vi "Initialize Close Variables.vi"(7 "Action":enum16{"Init", "Close"}(ring)=enum."Close", 8 "error in (no error)":errorcluster) -> (0 "error out":errorcluster)   [LabVIEW 2019]
uses:
  Controls/UDP - Event.ctl
  Controls/UDP - Status.ctl
  Controls/eFGV States.ctl
  Controls/FGV States.ctl
  Controls/Global - Device.vi
  Controls/Global - IP Address.vi
  Controls/Global - Done.vi
  Controls/Global - Comport.vi
  Controls/Global - Handle.vi
  Controls/Global - Unit.vi
  Controls/Global - ADC.vi
  Controls/Global - PID.vi
  Controls/Global - System.vi
  Controls/Global - Test.vi
  Controls/Global - Channel.vi
  Controls/Global - Data UDP.vi
  Controls/Global - Rendezvous.vi
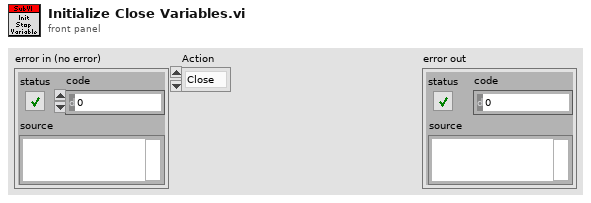
[diagram p1: front panel]
types:
  T1 = cluster{"Ch1":sgl, "Ch2":sgl, "Ch3":sgl, "Ch4":sgl, "Ch5":sgl, "Ch6":sgl, "Ch7":sgl, "Ch8":sgl, "Ch9":sgl, "Ch10":sgl, "Ch11":sgl, "Ch12":sgl, "Ch13":sgl, "Ch14":sgl, "Ch15":sgl, "Ch16":sgl}
  T2 = typedef "UDP - Event.ctl" = u16
  T3 = typedef "UDP - Status.ctl" = u16
  T4 = cluster{"Channels":cluster{"Ch1":sgl, "Ch2":sgl, "Ch3":sgl, "Ch4":sgl, "Ch5":sgl, "Ch6":sgl, "Ch7":sgl, "Ch8":sgl, "Ch9":sgl, "Ch10":sgl, "Ch11":sgl, "Ch12":sgl, "Ch13":sgl, "Ch14":sgl, "Ch15":sgl, "Ch16":sgl}, "Event":T2, "Status":T3, "IP":string}[]
  T5 = cluster{"Target Load":sgl, "Target Disp":sgl, "Rate":sgl, "Speed":sgl}[]
  T6 = cluster{"Out Type":u8, "Inverse":u8, "Monitor":u8, "Reserve":u8, "ACC Time":u32, "Pulse Rev":u32, "Stroke":u32, "Auto Off":u32, "Gear Ratio":sgl, "Pitch":sgl, "Max Speed":u32, "Jog Speed":u32, "Disp Coff":sgl, "Max Load":u32}[]
  T7 = cluster{"SP":sgl, "PV":sgl, "kP":sgl, "kI":sgl, "kD":sgl, "FF":sgl, "Err Band":sgl, "Max":i32, "Min":i32, "Ts":u32, "Out":i32, "Mode":u8}[]
  T8 = cluster{"Active Ch":u8[], "Filter Type":u8, "Post Filter":u8[], "Gain":u8[], "FS":u16, "IntOC":u8, "IntFC":u8, "SysOC":u8, "Cofficient":dbl[], "K":dbl[], "Max":i32}[]
  T9 = cluster{"Name":string[], "Unit":string[], "Decimal Point":u8[], "Ch Log":u8[], "H Alarm":u8[], "L Alarm":u8[], "H Limit":sgl[], "L Limit":sgl[], "Filter":u8[], "Gain":u8[], "Calib Type":u32[]}[]
  T10 = cluster{"IP Address":string, "port":string, "UDP ref":refnum<k16>}[]
  T11 = typedef "FGV States.ctl" = enum16{"Read", "Write"}
  T12 = typedef "eFGV States.ctl" = enum16{"Init", "Read", "Write", "Exit"}
  T13 = typedef "Rendezvous RefNum" = refnum<k1>
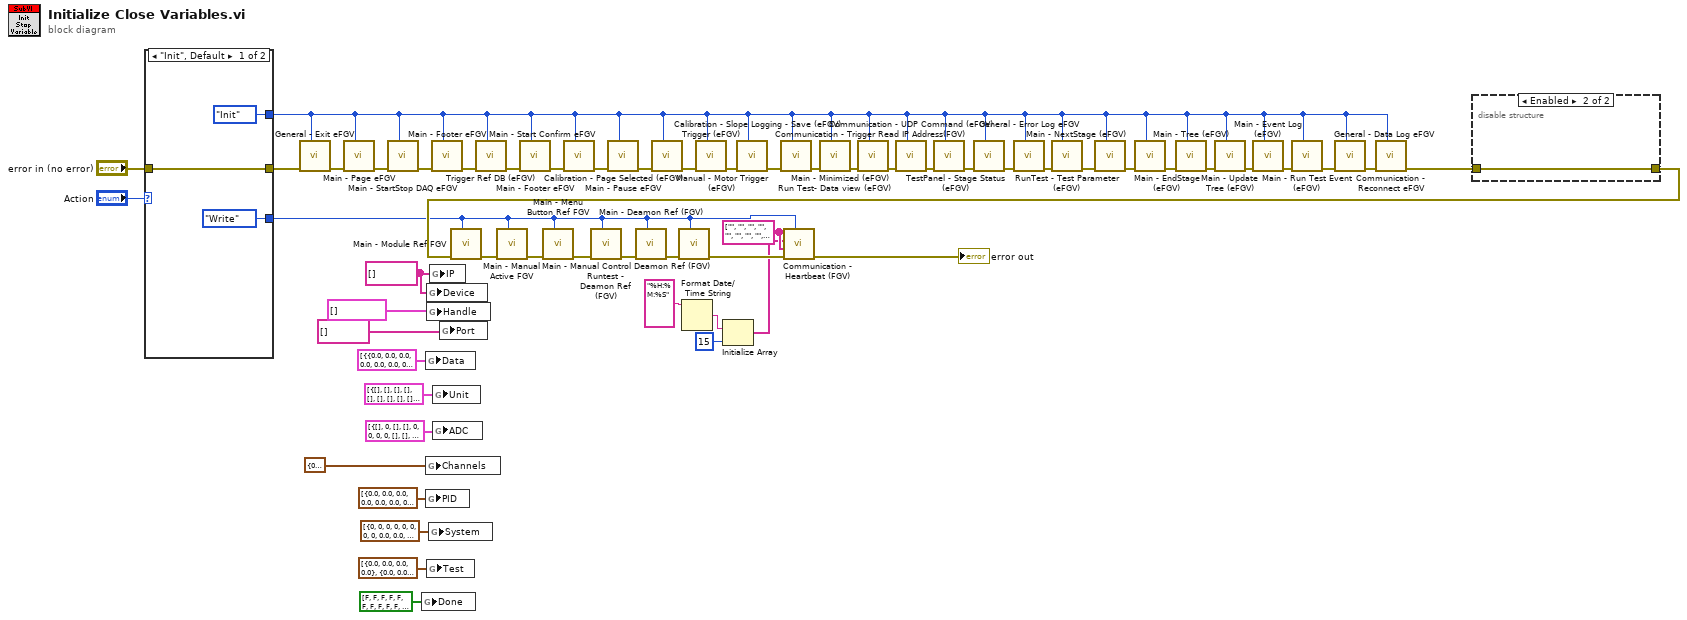
[diagram p0: block diagram]
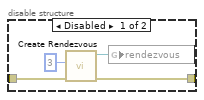
[diagram p2: hidden frame]
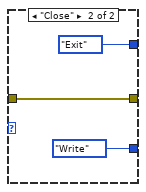
[diagram p3: hidden frame]
diagram:
  w10 = string[] ["", "", "", "", "", "", "", "", "", "", "", "", "", "", "", ""] ("IP")
  w35 = string[] [] ("SN")
  n1 = case shown="\"Init\", Default" "Action" {
    tunnel: [eFGV_States."Init" ("eFGV States") eFGV_States."Exit" ("eFGV States")] -> w1
    tunnel: [w58 w61] -> w55
    tunnel: "error in (no error)" -> [w58 w61]
    tunnel: [FGV_States."Write" ("Action") FGV_States."Write" ("Action")] -> w11
    frame "Init", Default {
    }
    frame "Close" {
    }
  }
  n2 = call "General - Exit eFGV.vi"("eFGV States"=w1, "error in (no error)"=w55) -> ("error out"=w48:errorcluster)  [unwired: 7 in, 2 out]
  n3 = call "Main - Page eFGV.vi"("eFGV States"=w1, "error in (no error)"=w48) -> ("error out"=w47:errorcluster)  [unwired: 7 in, 2 out]
  n4 = call "Main - StartStop DAQ eFGV.vi"("Action"=w1, "error in"=w47) -> ("error out"=w53:errorcluster)  [unwired: 7 in, 2 out]
  n5 = global write "Global - Done.vi" "Done"(bool[] [FALSE, FALSE, FALSE, FALSE, FALSE, FALSE, FALSE, FALSE, FALSE, FALSE, FALSE, FALSE, FALSE, FALSE, FALSE, FALSE] ("Done")) -> ()
  n6 = global write "Global - Channel.vi" "Data"(T4 [{"Channels"={"Ch1"=0.0, "Ch2"=0.0, "Ch3"=0.0, "Ch4"=0.0, "Ch5"=0.0, "Ch6"=0.0, "Ch7"=0.0, "Ch8"=0.0, "Ch9"=0.0, "Ch10"=0.0, "Ch11"=0.0, "Ch12"=0.0, "Ch13"=0.0, "Ch14"=0.0, "Ch15"=0.0, "Ch16"=0.0}, "Event"=0, "Status"=0, "IP"=""}, {"Channels"={"Ch1"=0.0, "Ch2"=0.0, "Ch3"=0.0, "Ch4"=0.0, "Ch5"=0.0, "Ch6"=0.0, "Ch7"=0.0, "Ch8"=0.0, "Ch9"=0.0, "Ch10"=0.0, "Ch11"=0.0, "Ch12"=0.0, "Ch13"=0.0, "Ch14"=0.0, "Ch15"=0.0, "Ch16"=0.0}, "Event"=0, "Status"=0, "IP"=""}, {"Channels"={"Ch1"=0.0, "Ch2"=0.0, "Ch3"=0.0, "Ch4"=0.0, "Ch5"=0.0, "Ch6"=0.0, "Ch7"=0.0, "Ch8"=0.0, "Ch9"=0.0, "Ch10"=0.0, "Ch11"=0.0, "Ch12"=0.0, "Ch13"=0.0, "Ch14"=0.0, "Ch15"=0.0, "Ch16"=0.0}, "Event"=0, "Status"=0, "IP"=""}, {"Channels"={"Ch1"=0.0, "Ch2"=0.0, "Ch3"=0.0, "Ch4"=0.0, "Ch5"=0.0, "Ch6"=0.0, "Ch7"=0.0, "Ch8"=0.0, "Ch9"=0.0, "Ch10"=0.0, "Ch11"=0.0, "Ch12"=0.0, "Ch13"=0.0, "Ch14"=0.0, "Ch15"=0.0, "Ch16"=0.0}, "Event"=0, "Status"=0, "IP"=""}, {"Channels"={"Ch1"=0.0, "Ch2"=0.0, "Ch3"=0.0, "Ch4"=0.0, "Ch5"=0.0, "Ch6"=0.0, "Ch7"=0.0, "Ch8"=0.0, "Ch9"=0.0, "Ch10"=0.0, "Ch11"=0.0, "Ch12"=0.0, "Ch13"=0.0, "Ch14"=0.0, "Ch15"=0.0, "Ch16"=0.0}, "Event"=0, "Status"=0, "IP"=""}, {"Channels"={"Ch1"=0.0, "Ch2"=0.0, "Ch3"=0.0, "Ch4"=0.0, "Ch5"=0.0, "Ch6"=0.0, "Ch7"=0.0, "Ch8"=0.0, "Ch9"=0.0, "Ch10"=0.0, "Ch11"=0.0, "Ch12"=0.0, "Ch13"=0.0, "Ch14"=0.0, "Ch15"=0.0, "Ch16"=0.0}, "Event"=0, "Status"=0, "IP"=""}, {"Channels"={"Ch1"=0.0, "Ch2"=0.0, "Ch3"=0.0, "Ch4"=0.0, "Ch5"=0.0, "Ch6"=0.0, "Ch7"=0.0, "Ch8"=0.0, "Ch9"=0.0, "Ch10"=0.0, "Ch11"=0.0, "Ch12"=0.0, "Ch13"=0.0, "Ch14"=0.0, "Ch15"=0.0, "Ch16"=0.0}, "Event"=0, "Status"=0, "IP"=""}, {"Channels"={"Ch1"=0.0, "Ch2"=0.0, "Ch3"=0.0, "Ch4"=0.0, "Ch5"=0.0, "Ch6"=0.0, "Ch7"=0.0, "Ch8"=0.0, "Ch9"=0.0, "Ch10"=0.0, "Ch11"=0.0, "Ch12"=0.0, "Ch13"=0.0, "Ch14"=0.0, "Ch15"=0.0, "Ch16"=0.0}, "Event"=0, "Status"=0, "IP"=""}, {"Channels"={"Ch1"=0.0, "Ch2"=0.0, "Ch3"=0.0, "Ch4"=0.0, "Ch5"=0.0, "Ch6"=0.0, "Ch7"=0.0, "Ch8"=0.0, "Ch9"=0.0, "Ch10"=0.0, "Ch11"=0.0, "Ch12"=0.0, "Ch13"=0.0, "Ch14"=0.0, "Ch15"=0.0, "Ch16"=0.0}, "Event"=0, "Status"=0, "IP"=""}, {"Channels"={"Ch1"=0.0, "Ch2"=0.0, "Ch3"=0.0, "Ch4"=0.0, "Ch5"=0.0, "Ch6"=0.0, "Ch7"=0.0, "Ch8"=0.0, "Ch9"=0.0, "Ch10"=0.0, "Ch11"=0.0, "Ch12"=0.0, "Ch13"=0.0, "Ch14"=0.0, "Ch15"=0.0, "Ch16"=0.0}, "Event"=0, "Status"=0, "IP"=""}, {"Channels"={"Ch1"=0.0, "Ch2"=0.0, "Ch3"=0.0, "Ch4"=0.0, "Ch5"=0.0, "Ch6"=0.0, "Ch7"=0.0, "Ch8"=0.0, "Ch9"=0.0, "Ch10"=0.0, "Ch11"=0.0, "Ch12"=0.0, "Ch13"=0.0, "Ch14"=0.0, "Ch15"=0.0, "Ch16"=0.0}, "Event"=0, "Status"=0, "IP"=""}, {"Channels"={"Ch1"=0.0, "Ch2"=0.0, "Ch3"=0.0, "Ch4"=0.0, "Ch5"=0.0, "Ch6"=0.0, "Ch7"=0.0, "Ch8"=0.0, "Ch9"=0.0, "Ch10"=0.0, "Ch11"=0.0, "Ch12"=0.0, "Ch13"=0.0, "Ch14"=0.0, "Ch15"=0.0, "Ch16"=0.0}, "Event"=0, "Status"=0, "IP"=""}, {"Channels"={"Ch1"=0.0, "Ch2"=0.0, "Ch3"=0.0, "Ch4"=0.0, "Ch5"=0.0, "Ch6"=0.0, "Ch7"=0.0, "Ch8"=0.0, "Ch9"=0.0, "Ch10"=0.0, "Ch11"=0.0, "Ch12"=0.0, "Ch13"=0.0, "Ch14"=0.0, "Ch15"=0.0, "Ch16"=0.0}, "Event"=0, "Status"=0, "IP"=""}, {"Channels"={"Ch1"=0.0, "Ch2"=0.0, "Ch3"=0.0, "Ch4"=0.0, "Ch5"=0.0, "Ch6"=0.0, "Ch7"=0.0, "Ch8"=0.0, "Ch9"=0.0, "Ch10"=0.0, "Ch11"=0.0, "Ch12"=0.0, "Ch13"=0.0, "Ch14"=0.0, "Ch15"=0.0, "Ch16"=0.0}, "Event"=0, "Status"=0, "IP"=""}, {"Channels"={"Ch1"=0.0, "Ch2"=0.0, "Ch3"=0.0, "Ch4"=0.0, "Ch5"=0.0, "Ch6"=0.0, "Ch7"=0.0, "Ch8"=0.0, "Ch9"=0.0, "Ch10"=0.0, "Ch11"=0.0, "Ch12"=0.0, "Ch13"=0.0, "Ch14"=0.0, "Ch15"=0.0, "Ch16"=0.0}, "Event"=0, "Status"=0, "IP"=""}, {"Channels"={"Ch1"=0.0, "Ch2"=0.0, "Ch3"=0.0, "Ch4"=0.0, "Ch5"=0.0, "Ch6"=0.0, "Ch7"=0.0, "Ch8"=0.0, "Ch9"=0.0, "Ch10"=0.0, "Ch11"=0.0, "Ch12"=0.0, "Ch13"=0.0, "Ch14"=0.0, "Ch15"=0.0, "Ch16"=0.0}, "Event"=0, "Status"=0, "IP"=""}] ("Data")) -> ()
  n7 = global write "Global - Data UDP.vi" "Channels"(T1 {"Ch1"=0.0, "Ch2"=0.0, "Ch3"=0.0, "Ch4"=0.0, "Ch5"=0.0, "Ch6"=0.0, "Ch7"=0.0, "Ch8"=0.0, "Ch9"=0.0, "Ch10"=0.0, "Ch11"=0.0, "Ch12"=0.0, "Ch13"=0.0, "Ch14"=0.0, "Ch15"=0.0, "Ch16"=0.0} ("Channels")) -> ()
  n8 = global write "Global - PID.vi" "PID"(T7 [{"SP"=0.0, "PV"=0.0, "kP"=0.0, "kI"=0.0, "kD"=0.0, "FF"=0.0, "Err Band"=0.0, "Max"=0, "Min"=0, "Ts"=0, "Out"=0, "Mode"=0}, {"SP"=0.0, "PV"=0.0, "kP"=0.0, "kI"=0.0, "kD"=0.0, "FF"=0.0, "Err Band"=0.0, "Max"=0, "Min"=0, "Ts"=0, "Out"=0, "Mode"=0}, {"SP"=0.0, "PV"=0.0, "kP"=0.0, "kI"=0.0, "kD"=0.0, "FF"=0.0, "Err Band"=0.0, "Max"=0, "Min"=0, "Ts"=0, "Out"=0, "Mode"=0}, {"SP"=0.0, "PV"=0.0, "kP"=0.0, "kI"=0.0, "kD"=0.0, "FF"=0.0, "Err Band"=0.0, "Max"=0, "Min"=0, "Ts"=0, "Out"=0, "Mode"=0}, {"SP"=0.0, "PV"=0.0, "kP"=0.0, "kI"=0.0, "kD"=0.0, "FF"=0.0, "Err Band"=0.0, "Max"=0, "Min"=0, "Ts"=0, "Out"=0, "Mode"=0}, {"SP"=0.0, "PV"=0.0, "kP"=0.0, "kI"=0.0, "kD"=0.0, "FF"=0.0, "Err Band"=0.0, "Max"=0, "Min"=0, "Ts"=0, "Out"=0, "Mode"=0}, {"SP"=0.0, "PV"=0.0, "kP"=0.0, "kI"=0.0, "kD"=0.0, "FF"=0.0, "Err Band"=0.0, "Max"=0, "Min"=0, "Ts"=0, "Out"=0, "Mode"=0}, {"SP"=0.0, "PV"=0.0, "kP"=0.0, "kI"=0.0, "kD"=0.0, "FF"=0.0, "Err Band"=0.0, "Max"=0, "Min"=0, "Ts"=0, "Out"=0, "Mode"=0}, {"SP"=0.0, "PV"=0.0, "kP"=0.0, "kI"=0.0, "kD"=0.0, "FF"=0.0, "Err Band"=0.0, "Max"=0, "Min"=0, "Ts"=0, "Out"=0, "Mode"=0}, {"SP"=0.0, "PV"=0.0, "kP"=0.0, "kI"=0.0, "kD"=0.0, "FF"=0.0, "Err Band"=0.0, "Max"=0, "Min"=0, "Ts"=0, "Out"=0, "Mode"=0}, {"SP"=0.0, "PV"=0.0, "kP"=0.0, "kI"=0.0, "kD"=0.0, "FF"=0.0, "Err Band"=0.0, "Max"=0, "Min"=0, "Ts"=0, "Out"=0, "Mode"=0}, {"SP"=0.0, "PV"=0.0, "kP"=0.0, "kI"=0.0, "kD"=0.0, "FF"=0.0, "Err Band"=0.0, "Max"=0, "Min"=0, "Ts"=0, "Out"=0, "Mode"=0}, {"SP"=0.0, "PV"=0.0, "kP"=0.0, "kI"=0.0, "kD"=0.0, "FF"=0.0, "Err Band"=0.0, "Max"=0, "Min"=0, "Ts"=0, "Out"=0, "Mode"=0}, {"SP"=0.0, "PV"=0.0, "kP"=0.0, "kI"=0.0, "kD"=0.0, "FF"=0.0, "Err Band"=0.0, "Max"=0, "Min"=0, "Ts"=0, "Out"=0, "Mode"=0}, {"SP"=0.0, "PV"=0.0, "kP"=0.0, "kI"=0.0, "kD"=0.0, "FF"=0.0, "Err Band"=0.0, "Max"=0, "Min"=0, "Ts"=0, "Out"=0, "Mode"=0}, {"SP"=0.0, "PV"=0.0, "kP"=0.0, "kI"=0.0, "kD"=0.0, "FF"=0.0, "Err Band"=0.0, "Max"=0, "Min"=0, "Ts"=0, "Out"=0, "Mode"=0}] ("PID")) -> ()
  n9 = global write "Global - Device.vi" "Device"(w35) -> ()
  n10 = global write "Global - Handle.vi" "Handle"(T10 [] ("Handle")) -> ()
  n11 = global write "Global - Test.vi" "Test"(T5 [{"Target Load"=0.0, "Target Disp"=0.0, "Rate"=0.0, "Speed"=0.0}, {"Target Load"=0.0, "Target Disp"=0.0, "Rate"=0.0, "Speed"=0.0}, {"Target Load"=0.0, "Target Disp"=0.0, "Rate"=0.0, "Speed"=0.0}, {"Target Load"=0.0, "Target Disp"=0.0, "Rate"=0.0, "Speed"=0.0}, {"Target Load"=0.0, "Target Disp"=0.0, "Rate"=0.0, "Speed"=0.0}, {"Target Load"=0.0, "Target Disp"=0.0, "Rate"=0.0, "Speed"=0.0}, {"Target Load"=0.0, "Target Disp"=0.0, "Rate"=0.0, "Speed"=0.0}, {"Target Load"=0.0, "Target Disp"=0.0, "Rate"=0.0, "Speed"=0.0}, {"Target Load"=0.0, "Target Disp"=0.0, "Rate"=0.0, "Speed"=0.0}, {"Target Load"=0.0, "Target Disp"=0.0, "Rate"=0.0, "Speed"=0.0}, {"Target Load"=0.0, "Target Disp"=0.0, "Rate"=0.0, "Speed"=0.0}, {"Target Load"=0.0, "Target Disp"=0.0, "Rate"=0.0, "Speed"=0.0}, {"Target Load"=0.0, "Target Disp"=0.0, "Rate"=0.0, "Speed"=0.0}, {"Target Load"=0.0, "Target Disp"=0.0, "Rate"=0.0, "Speed"=0.0}, {"Target Load"=0.0, "Target Disp"=0.0, "Rate"=0.0, "Speed"=0.0}, {"Target Load"=0.0, "Target Disp"=0.0, "Rate"=0.0, "Speed"=0.0}] ("Test")) -> ()
  n12 = global write "Global - System.vi" "System"(T6 [{"Out Type"=0, "Inverse"=0, "Monitor"=0, "Reserve"=0, "ACC Time"=0, "Pulse Rev"=0, "Stroke"=0, "Auto Off"=0, "Gear Ratio"=0.0, "Pitch"=0.0, "Max Speed"=0, "Jog Speed"=0, "Disp Coff"=0.0, "Max Load"=0}, {"Out Type"=0, "Inverse"=0, "Monitor"=0, "Reserve"=0, "ACC Time"=0, "Pulse Rev"=0, "Stroke"=0, "Auto Off"=0, "Gear Ratio"=0.0, "Pitch"=0.0, "Max Speed"=0, "Jog Speed"=0, "Disp Coff"=0.0, "Max Load"=0}, {"Out Type"=0, "Inverse"=0, "Monitor"=0, "Reserve"=0, "ACC Time"=0, "Pulse Rev"=0, "Stroke"=0, "Auto Off"=0, "Gear Ratio"=0.0, "Pitch"=0.0, "Max Speed"=0, "Jog Speed"=0, "Disp Coff"=0.0, "Max Load"=0}, {"Out Type"=0, "Inverse"=0, "Monitor"=0, "Reserve"=0, "ACC Time"=0, "Pulse Rev"=0, "Stroke"=0, "Auto Off"=0, "Gear Ratio"=0.0, "Pitch"=0.0, "Max Speed"=0, "Jog Speed"=0, "Disp Coff"=0.0, "Max Load"=0}, {"Out Type"=0, "Inverse"=0, "Monitor"=0, "Reserve"=0, "ACC Time"=0, "Pulse Rev"=0, "Stroke"=0, "Auto Off"=0, "Gear Ratio"=0.0, "Pitch"=0.0, "Max Speed"=0, "Jog Speed"=0, "Disp Coff"=0.0, "Max Load"=0}, {"Out Type"=0, "Inverse"=0, "Monitor"=0, "Reserve"=0, "ACC Time"=0, "Pulse Rev"=0, "Stroke"=0, "Auto Off"=0, "Gear Ratio"=0.0, "Pitch"=0.0, "Max Speed"=0, "Jog Speed"=0, "Disp Coff"=0.0, "Max Load"=0}, {"Out Type"=0, "Inverse"=0, "Monitor"=0, "Reserve"=0, "ACC Time"=0, "Pulse Rev"=0, "Stroke"=0, "Auto Off"=0, "Gear Ratio"=0.0, "Pitch"=0.0, "Max Speed"=0, "Jog Speed"=0, "Disp Coff"=0.0, "Max Load"=0}, {"Out Type"=0, "Inverse"=0, "Monitor"=0, "Reserve"=0, "ACC Time"=0, "Pulse Rev"=0, "Stroke"=0, "Auto Off"=0, "Gear Ratio"=0.0, "Pitch"=0.0, "Max Speed"=0, "Jog Speed"=0, "Disp Coff"=0.0, "Max Load"=0}, {"Out Type"=0, "Inverse"=0, "Monitor"=0, "Reserve"=0, "ACC Time"=0, "Pulse Rev"=0, "Stroke"=0, "Auto Off"=0, "Gear Ratio"=0.0, "Pitch"=0.0, "Max Speed"=0, "Jog Speed"=0, "Disp Coff"=0.0, "Max Load"=0}, {"Out Type"=0, "Inverse"=0, "Monitor"=0, "Reserve"=0, "ACC Time"=0, "Pulse Rev"=0, "Stroke"=0, "Auto Off"=0, "Gear Ratio"=0.0, "Pitch"=0.0, "Max Speed"=0, "Jog Speed"=0, "Disp Coff"=0.0, "Max Load"=0}, {"Out Type"=0, "Inverse"=0, "Monitor"=0, "Reserve"=0, "ACC Time"=0, "Pulse Rev"=0, "Stroke"=0, "Auto Off"=0, "Gear Ratio"=0.0, "Pitch"=0.0, "Max Speed"=0, "Jog Speed"=0, "Disp Coff"=0.0, "Max Load"=0}, {"Out Type"=0, "Inverse"=0, "Monitor"=0, "Reserve"=0, "ACC Time"=0, "Pulse Rev"=0, "Stroke"=0, "Auto Off"=0, "Gear Ratio"=0.0, "Pitch"=0.0, "Max Speed"=0, "Jog Speed"=0, "Disp Coff"=0.0, "Max Load"=0}, {"Out Type"=0, "Inverse"=0, "Monitor"=0, "Reserve"=0, "ACC Time"=0, "Pulse Rev"=0, "Stroke"=0, "Auto Off"=0, "Gear Ratio"=0.0, "Pitch"=0.0, "Max Speed"=0, "Jog Speed"=0, "Disp Coff"=0.0, "Max Load"=0}, {"Out Type"=0, "Inverse"=0, "Monitor"=0, "Reserve"=0, "ACC Time"=0, "Pulse Rev"=0, "Stroke"=0, "Auto Off"=0, "Gear Ratio"=0.0, "Pitch"=0.0, "Max Speed"=0, "Jog Speed"=0, "Disp Coff"=0.0, "Max Load"=0}, {"Out Type"=0, "Inverse"=0, "Monitor"=0, "Reserve"=0, "ACC Time"=0, "Pulse Rev"=0, "Stroke"=0, "Auto Off"=0, "Gear Ratio"=0.0, "Pitch"=0.0, "Max Speed"=0, "Jog Speed"=0, "Disp Coff"=0.0, "Max Load"=0}, {"Out Type"=0, "Inverse"=0, "Monitor"=0, "Reserve"=0, "ACC Time"=0, "Pulse Rev"=0, "Stroke"=0, "Auto Off"=0, "Gear Ratio"=0.0, "Pitch"=0.0, "Max Speed"=0, "Jog Speed"=0, "Disp Coff"=0.0, "Max Load"=0}] ("System")) -> ()
  n13 = global write "Global - IP Address.vi" "IP"(w35) -> ()
  n14 = call "Main - Footer eFGV.vi"("Action"=w1, "error in"=w53) -> ("error out"=w46:errorcluster)  [unwired: 7 in, 2 out]
  n15 = global write "Global - Unit.vi" "Unit"(T9 [{"Name"=[], "Unit"=[], "Decimal Point"=[], "Ch Log"=[], "H Alarm"=[], "L Alarm"=[], "H Limit"=[], "L Limit"=[], "Filter"=[], "Gain"=[], "Calib Type"=[]}, {"Name"=[], "Unit"=[], "Decimal Point"=[], "Ch Log"=[], "H Alarm"=[], "L Alarm"=[], "H Limit"=[], "L Limit"=[], "Filter"=[], "Gain"=[], "Calib Type"=[]}, {"Name"=[], "Unit"=[], "Decimal Point"=[], "Ch Log"=[], "H Alarm"=[], "L Alarm"=[], "H Limit"=[], "L Limit"=[], "Filter"=[], "Gain"=[], "Calib Type"=[]}, {"Name"=[], "Unit"=[], "Decimal Point"=[], "Ch Log"=[], "H Alarm"=[], "L Alarm"=[], "H Limit"=[], "L Limit"=[], "Filter"=[], "Gain"=[], "Calib Type"=[]}, {"Name"=[], "Unit"=[], "Decimal Point"=[], "Ch Log"=[], "H Alarm"=[], "L Alarm"=[], "H Limit"=[], "L Limit"=[], "Filter"=[], "Gain"=[], "Calib Type"=[]}, {"Name"=[], "Unit"=[], "Decimal Point"=[], "Ch Log"=[], "H Alarm"=[], "L Alarm"=[], "H Limit"=[], "L Limit"=[], "Filter"=[], "Gain"=[], "Calib Type"=[]}, {"Name"=[], "Unit"=[], "Decimal Point"=[], "Ch Log"=[], "H Alarm"=[], "L Alarm"=[], "H Limit"=[], "L Limit"=[], "Filter"=[], "Gain"=[], "Calib Type"=[]}, {"Name"=[], "Unit"=[], "Decimal Point"=[], "Ch Log"=[], "H Alarm"=[], "L Alarm"=[], "H Limit"=[], "L Limit"=[], "Filter"=[], "Gain"=[], "Calib Type"=[]}, {"Name"=[], "Unit"=[], "Decimal Point"=[], "Ch Log"=[], "H Alarm"=[], "L Alarm"=[], "H Limit"=[], "L Limit"=[], "Filter"=[], "Gain"=[], "Calib Type"=[]}, {"Name"=[], "Unit"=[], "Decimal Point"=[], "Ch Log"=[], "H Alarm"=[], "L Alarm"=[], "H Limit"=[], "L Limit"=[], "Filter"=[], "Gain"=[], "Calib Type"=[]}, {"Name"=[], "Unit"=[], "Decimal Point"=[], "Ch Log"=[], "H Alarm"=[], "L Alarm"=[], "H Limit"=[], "L Limit"=[], "Filter"=[], "Gain"=[], "Calib Type"=[]}, {"Name"=[], "Unit"=[], "Decimal Point"=[], "Ch Log"=[], "H Alarm"=[], "L Alarm"=[], "H Limit"=[], "L Limit"=[], "Filter"=[], "Gain"=[], "Calib Type"=[]}, {"Name"=[], "Unit"=[], "Decimal Point"=[], "Ch Log"=[], "H Alarm"=[], "L Alarm"=[], "H Limit"=[], "L Limit"=[], "Filter"=[], "Gain"=[], "Calib Type"=[]}, {"Name"=[], "Unit"=[], "Decimal Point"=[], "Ch Log"=[], "H Alarm"=[], "L Alarm"=[], "H Limit"=[], "L Limit"=[], "Filter"=[], "Gain"=[], "Calib Type"=[]}, {"Name"=[], "Unit"=[], "Decimal Point"=[], "Ch Log"=[], "H Alarm"=[], "L Alarm"=[], "H Limit"=[], "L Limit"=[], "Filter"=[], "Gain"=[], "Calib Type"=[]}, {"Name"=[], "Unit"=[], "Decimal Point"=[], "Ch Log"=[], "H Alarm"=[], "L Alarm"=[], "H Limit"=[], "L Limit"=[], "Filter"=[], "Gain"=[], "Calib Type"=[]}] ("Unit")) -> ()
  n16 = global write "Global - ADC.vi" "ADC"(T8 [{"Active Ch"=[], "Filter Type"=0, "Post Filter"=[], "Gain"=[], "FS"=0, "IntOC"=0, "IntFC"=0, "SysOC"=0, "Cofficient"=[], "K"=[], "Max"=0}, {"Active Ch"=[], "Filter Type"=0, "Post Filter"=[], "Gain"=[], "FS"=0, "IntOC"=0, "IntFC"=0, "SysOC"=0, "Cofficient"=[], "K"=[], "Max"=0}, {"Active Ch"=[], "Filter Type"=0, "Post Filter"=[], "Gain"=[], "FS"=0, "IntOC"=0, "IntFC"=0, "SysOC"=0, "Cofficient"=[], "K"=[], "Max"=0}, {"Active Ch"=[], "Filter Type"=0, "Post Filter"=[], "Gain"=[], "FS"=0, "IntOC"=0, "IntFC"=0, "SysOC"=0, "Cofficient"=[], "K"=[], "Max"=0}, {"Active Ch"=[], "Filter Type"=0, "Post Filter"=[], "Gain"=[], "FS"=0, "IntOC"=0, "IntFC"=0, "SysOC"=0, "Cofficient"=[], "K"=[], "Max"=0}, {"Active Ch"=[], "Filter Type"=0, "Post Filter"=[], "Gain"=[], "FS"=0, "IntOC"=0, "IntFC"=0, "SysOC"=0, "Cofficient"=[], "K"=[], "Max"=0}, {"Active Ch"=[], "Filter Type"=0, "Post Filter"=[], "Gain"=[], "FS"=0, "IntOC"=0, "IntFC"=0, "SysOC"=0, "Cofficient"=[], "K"=[], "Max"=0}, {"Active Ch"=[], "Filter Type"=0, "Post Filter"=[], "Gain"=[], "FS"=0, "IntOC"=0, "IntFC"=0, "SysOC"=0, "Cofficient"=[], "K"=[], "Max"=0}, {"Active Ch"=[], "Filter Type"=0, "Post Filter"=[], "Gain"=[], "FS"=0, "IntOC"=0, "IntFC"=0, "SysOC"=0, "Cofficient"=[], "K"=[], "Max"=0}, {"Active Ch"=[], "Filter Type"=0, "Post Filter"=[], "Gain"=[], "FS"=0, "IntOC"=0, "IntFC"=0, "SysOC"=0, "Cofficient"=[], "K"=[], "Max"=0}, {"Active Ch"=[], "Filter Type"=0, "Post Filter"=[], "Gain"=[], "FS"=0, "IntOC"=0, "IntFC"=0, "SysOC"=0, "Cofficient"=[], "K"=[], "Max"=0}, {"Active Ch"=[], "Filter Type"=0, "Post Filter"=[], "Gain"=[], "FS"=0, "IntOC"=0, "IntFC"=0, "SysOC"=0, "Cofficient"=[], "K"=[], "Max"=0}, {"Active Ch"=[], "Filter Type"=0, "Post Filter"=[], "Gain"=[], "FS"=0, "IntOC"=0, "IntFC"=0, "SysOC"=0, "Cofficient"=[], "K"=[], "Max"=0}, {"Active Ch"=[], "Filter Type"=0, "Post Filter"=[], "Gain"=[], "FS"=0, "IntOC"=0, "IntFC"=0, "SysOC"=0, "Cofficient"=[], "K"=[], "Max"=0}, {"Active Ch"=[], "Filter Type"=0, "Post Filter"=[], "Gain"=[], "FS"=0, "IntOC"=0, "IntFC"=0, "SysOC"=0, "Cofficient"=[], "K"=[], "Max"=0}, {"Active Ch"=[], "Filter Type"=0, "Post Filter"=[], "Gain"=[], "FS"=0, "IntOC"=0, "IntFC"=0, "SysOC"=0, "Cofficient"=[], "K"=[], "Max"=0}] ("ADC")) -> ()
  n17 = global write "Global - Comport.vi" "Port"(string[] [] ("Comport")) -> ()
  n18 = call "Trigger Ref DB (eFGV).vi"("Action"=w1, "error in"=w46) -> ("error out"=w45:errorcluster)  [unwired: 7 in, 2 out]
  n19 = call "Main - Footer eFGV.vi"("Action"=w1, "error in"=w45) -> ("error out"=w50:errorcluster)  [unwired: 7 in, 2 out]
  n20 = call "Main - Start Confirm eFGV.vi"("Action"=w1, "error in"=w50) -> ("error out"=w49:errorcluster)  [unwired: 7 in, 2 out]
  n21 = call "Main - Pause eFGV.vi"("Action"=w1, "error in"=w49) -> ("error out"=w44:errorcluster)  [unwired: 7 in, 2 out]
  n22 = call "Calibration - Page Selected (eFGV).vi"("Action"=w1, "error in"=w44) -> ("error out"=w43:errorcluster)  [unwired: 7 in, 2 out]
  n23 = Format Date/Time String(time format string (%c)="%H:%M:%S") -> (date/time string=w8:string)  [unwired: 2 in]
  n24 = call "Calibration - Slope Trigger (eFGV).vi"("Action"=w1, "error in"=w43) -> ("error out"=w40:errorcluster)  [unwired: 7 in, 2 out]
  n25 = Initialize Array(w8, 15 ("dimension size")) -> (w6:string[])
  n26 = call "Manual - Motor Trigger (eFGV).vi"("Action"=w1, "error in"=w40) -> ("error out"=w39:errorcluster)  [unwired: 7 in, 2 out]
  n27 = call "Logging - Save (eFGV).vi"("Action"=w1, "error in"=w39) -> ("error out"=w42:errorcluster)  [unwired: 7 in, 2 out]
  n28 = call "Run Test- Data view (eFGV).vi"("eFGV States"=w1, "error in (no error)"=w42) -> ("error out"=w38:errorcluster)  [unwired: 7 in, 2 out]
  n29 = call "Main - Minimized (eFGV).vi"("Action"=w1, "error in"=w38) -> ("error out"=w41:errorcluster)  [unwired: 7 in, 2 out]
  n30 = call "Communication - UDP Command (eFGV).vi"("Action"=w1, "error in"=w41) -> ("error out"=w37:errorcluster)  [unwired: 7 in, 2 out]
  n31 = call "Communication - Trigger Read IP Address(FGV).vi"("Action"=w1, "error in"=w37) -> ("error out"=w36:errorcluster)  [unwired: 7 in, 2 out]
  n32 = call "TestPanel - Stage Status (eFGV).vi"("Action"=w1, "error in"=w36) -> ("error out"=w32:errorcluster)  [unwired: 7 in, 2 out]
  n33 = call "General - Error Log eFGV.vi"("eFGV States"=w1, "error in (no error)"=w32) -> ("error out"=w21:errorcluster)  [unwired: 7 in, 2 out]
  n34 = call "RunTest - Test Parameter (eFGV).vi"("Action"=w1, "error in"=w21) -> ("error out"=w20:errorcluster)  [unwired: 7 in, 2 out]
  n35 = call "Main - NextStage (eFGV).vi"("Action"=w1, "error in"=w20) -> ("error out"=w30:errorcluster)  [unwired: 7 in, 2 out]
  n36 = call "Main - EndStage (eFGV).vi"("Action"=w1, "error in"=w30) -> ("error out"=w23:errorcluster)  [unwired: 7 in, 2 out]
  n37 = call "Main - Tree (eFGV).vi"("Action"=w1, "error in"=w23) -> ("error out"=w22:errorcluster)  [unwired: 7 in, 2 out]
  n38 = call "Main - Update Tree (eFGV).vi"("Action"=w1, "error in"=w22) -> ("error out"=w16:errorcluster)  [unwired: 7 in, 2 out]
  n39 = call "Main - Event Log (eFGV).vi"("Action"=w1, "error in"=w16) -> ("error out"=w5:errorcluster)  [unwired: 6 in, 3 out]
  n40 = call "Main - Run Test Event (eFGV).vi"("Action"=w1, "error in"=w5) -> ("error out"=w4:errorcluster)  [unwired: 7 in, 2 out]
  n41 = call "General - Data Log eFGV.vi"("eFGV States"=w1, "error in (no error)"=w4) -> ("error out"=w3:errorcluster)  [unwired: 7 in, 2 out]
  n42 = call "Communication - Reconnect eFGV.vi"("eFGV States"=w1, "error in (no error)"=w3) -> ("error out"=w2:errorcluster)  [unwired: 7 in, 2 out]
  n43 = disable-structure shown="Enabled" {
    disable-tunnel: [w64 w67] -> w31
    disable-tunnel: w2 -> [w63 w67]
    frame Disabled {
      n44 = call <vilib>:"Create Rendezvous.vi"("error in (no error)"=w63, "size (2)"=3) -> ("error out"=w64:errorcluster, "rendezvous"=w65:T13)  [unwired: 3 in, 1 out]
      n45 = global write "Global - Rendezvous.vi" "rendezvous"(w65) -> ()
    }
    frame Enabled {
    }
  }
  n46 = call "Main - Module Ref FGV.vi"("Action"=w11, "error In"=w31) -> ("error out"=w51:errorcluster)  [unwired: 7 in, 2 out]
  n47 = call "Main - Manual Active FGV.vi"("Action"=w11, "error In"=w51) -> ("error out"=w52:errorcluster)  [unwired: 6 in, 3 out]
  n48 = call "Main - Menu Button Ref FGV.vi"("Action"=w11, "error In"=w52) -> ("error out"=w19:errorcluster)  [unwired: 8 in, 1 out]
  n49 = call "Runtest - Deamon Ref (FGV).vi"("Action"=w11, "error in"=w19) -> ("error out"=w18:errorcluster)  [unwired: 7 in, 2 out]
  n50 = call "Main - Deamon Ref (FGV).vi"("Action"=w11, "error in"=w18) -> ("error out"=w17:errorcluster)  [unwired: 8 in, 1 out]
  n51 = call "Main - Manual Control Deamon Ref (FGV).vi"("Action"=w11, "error in"=w17) -> ("error out"=w13:errorcluster)  [unwired: 7 in, 2 out]
  n52 = call "Communication - Heartbeat (FGV).vi"("Action"=w11, "error in (no error)"=w13, "Previous"=w10, "Timestamp"=w6, "IP"=w10) -> ("error out"=→"error out":errorcluster)  [unwired: 3 in, 3 out]
